vi "MoveClassOnDisk.vi"(8 "error in (no error)":errorcluster, 9 "NewName":string, 10 "NewPath":path, 11 "LVClassLibrary Refnum":refnum<vi>) -> (0 "error out":errorcluster, 3 "Library Refnum out":refnum<vi>)   [LabVIEW 2014, in "ClassRenamer.lvclass"]
uses:
  ClassRenamer.lvclass
  <vilib>/Utility/EditLVLibs/Edit LVLibs.lvlib
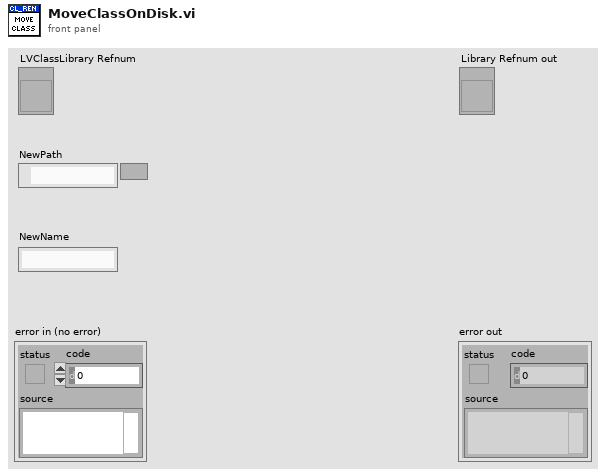
[diagram p1: front panel]
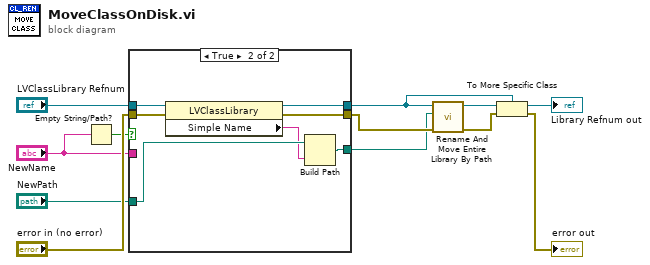
[diagram p0: block diagram]
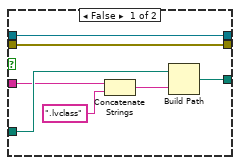
[diagram p2: hidden frame]
diagram:
  n1 = Empty String/Path?(string/path="NewName") -> (empty?=w8:bool)
  n2 = case shown="True" w8 {
    tunnel: "LVClassLibrary Refnum" -> [w19 w26]
    tunnel: "NewName" -> [w15 _]
    tunnel: "NewPath" -> [w17 w24]
    tunnel: [w19 w25] -> w1
    tunnel: "error in (no error)" -> [w18 w22]
    tunnel: [w18 w21] -> w5
    tunnel: [w16 w20] -> w4
    frame False {
      n3 = Concatenate Strings(w15, ".lvclass" ("string")) -> (w14:string)
      n4 = Build Path(base path=w17, name or relative path=w14) -> (appended path=w16:path)
    }
    frame True {
      n5 = property class="LVClassLibrary"(reference=w26, error in=w22) -> (reference out=w25:refnum<vi>, error out=w21:errorcluster, "Simple Name"=w23:string)
      n6 = Build Path(base path=w24, name or relative path=w23) -> (appended path=w20:path)
    }
  }
  n7 = call <vilib>:"Rename And Move Entire Library By Path.vi"("error in (no error)"=w5, "New library path"=w4, "Library ref in"=w1) -> ("error out"=w2:errorcluster, "Library ref out"=w3:refnum<vi>)  [unwired: 7 in]
  n8 = To More Specific Class(target class=w1, reference=w3, error in=w2) -> (specific class reference=→"Library Refnum out":refnum<vi>, error out=→"error out":errorcluster)
